vi "Motor Calibrator.vi"() -> ()   [LabVIEW 2013]
doc: "<B>Motor Control.vi</B> demonstrates simplistic control of a motor using PWM."
uses:
  <vilib>/Rock Robotics/SystemInterfaces/Typedef/FPGA_TypedefDigitalModule.ctl
  <vilib>/Rock Robotics/WPI/MotorControl/WPI_MotorControlOpen Victor.vi
  <vilib>/Rock Robotics/WPI/MotorControl/WPI_MotorControlOpen Jaguar.vi
  <vilib>/Rock Robotics/WPI/MotorControl/WPI_MotorControlOpen Talon.vi
panel:
  in  "Next":bool
  out "Current Motor":string="None"
  out "Motor Output":dbl(slide) scale=-1.0..1.0
  in  "Motor Controllers":cluster{"Type":u16, "PWM":string}[](array[cluster])=[{"Type"=0, "PWM"="PWM 1"}, {"Type"=0, "PWM"="PWM 2"}, {"Type"=0, "PWM"="PWM 3"}, {"Type"=0, "PWM"="PWM 4"}, {"Type"=0, "PWM"="PWM 5"}, {"Type"=0, "PWM"="PWM 6"}, {"Type"=0, "PWM"="PWM 7"}, {"Type"=0, "PWM"="PWM 8"}, {"Type"=0, "PWM"="PWM 9"}, {"Type"=0, "PWM"="PWM 10"}] {"Type" items=["Disabled", "Victor", "Jaguar", "Talon"]}
  in  "DIO Module":T1
  # "Calibration Instructions"
  # "Victor 888\n\n1. Power ON the speed controller.\n2. Press and hold the Cal button. After a moment, the LED indicator on the Victor will begin alternating between \n    RED and GREEN to indicate a cal mode.\n3. While continuing to hold the Cal button, move the joystick to the maximum and minimum positions. \n    This can be done in any order and as many times as desired.\n4. While continuing to hold the Cal button, return the joystick to center (neutral position).\n5. Release the Cal button.\n6. A flashing GREEN indicator confirms a successful calibration.\n7. A flashing RED indicator denotes an unsuccessful calibration.\n    An unsuccessful calibration occurs when either:\n    a) Insufficient joystick travel was detected in forward and/or reverse.\n    b) The trim tab is too far from center.\n    c) The Joystick is too far from center when Cal is released."
  # "Jaguar\n\n1. Hold down the USER switch with a straightened paper clip for 5 seconds.\n2. The LED flashes Red and Green to indicate Calibration mode.\n3. Instruct the controller to send a full-forward signal for one or more seconds.\n4. Instruct the controller to send a full-reverse signal for one or more seconds.\n5. The LED flashes Green and Yellow quickly to indicate a successful calibration."
  # "Talon\n\n1. Press and hold the button labeled “CAL” with a paper clip. The LED should begin to blink red/green. \n2. Continue to keep the button pressed while moving the joystick full forward and full reverse. \n    You may do this as many times as you like. \n3. Center the joystick and then release the CAL button. \n4. If calibration was successful, the LED will blink green several times. If the LED blinks red several times,\n    the calibration was not valid. If this happens, the Talon will use the last valid calibration values."
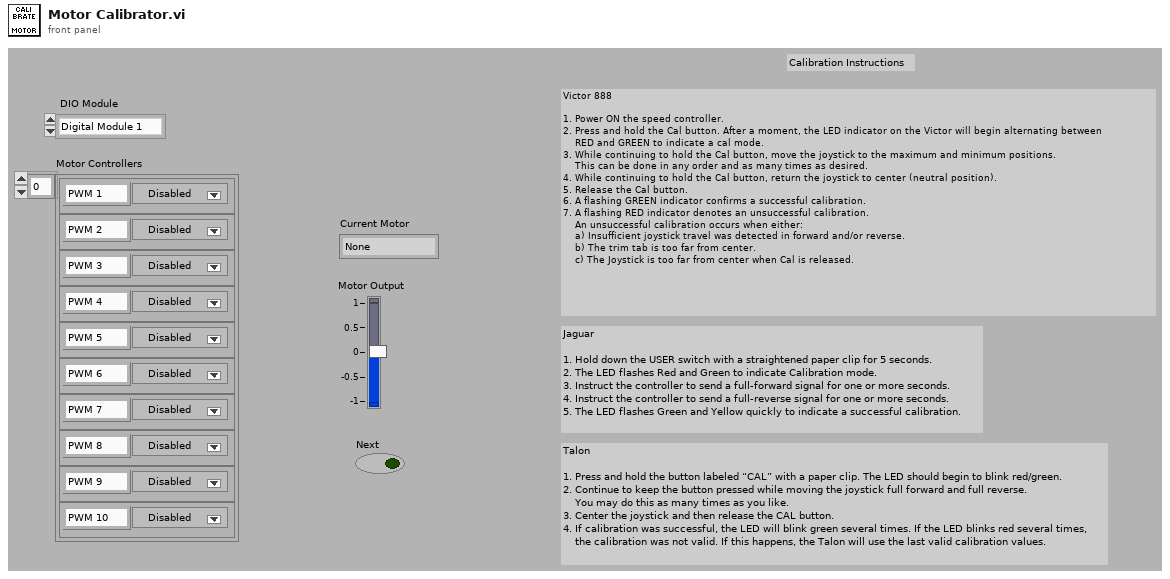
[diagram p1: front panel]
types:
  T1 = typedef "FPGA_TypedefDigitalModule.ctl" = enum16{"Digital Module 1", "Digital Module 2"}
  T2 = typedef "WPI_MotorControlDeviceRef.ctl" = cluster{"DeviceStatus":errorcluster, "Type":enum16{"PWM", "CAN"}, "PWM":cluster{"Digital Module":T1, "PWM Channel":T3, "DeadBand":T4}, "CAN":cluster{"Device Number":u8, "Control Mode":T5, "Semaphore":T6, "Max Vout":dbl}, "Invert":bool, "TransformRef":T7, "InvTransformRef":T7}
  T3 = typedef "FPGA_DIOPWMChannel.ctl" = enum8{"PWM 1", "PWM 2", "PWM 3", "PWM 4", "PWM 5", "PWM 6", "PWM 7", "PWM 8", "PWM 9", "PWM 10", "Invalid"}
  T4 = typedef "WPI_PWMDeadband.ctl" = cluster{"Name":string, "maxPositivePwm":i32, "minPositivePwm":i32, "centerPwm":i32, "maxNegativePwm":i32, "minNegativePwm":i32, "angularRange":u16}
  T5 = typedef "WPI_CANJaguar_ControlMode.ctl" = enum8{"Percent VBus", "Current", "Speed", "Position", "Voltage"}
  T6 = typedef "Semaphore RefNum" = refnum<k1>
  T7 = typedef "WPI_PWMTransform_ConPane.ctl" = refnum<vi>
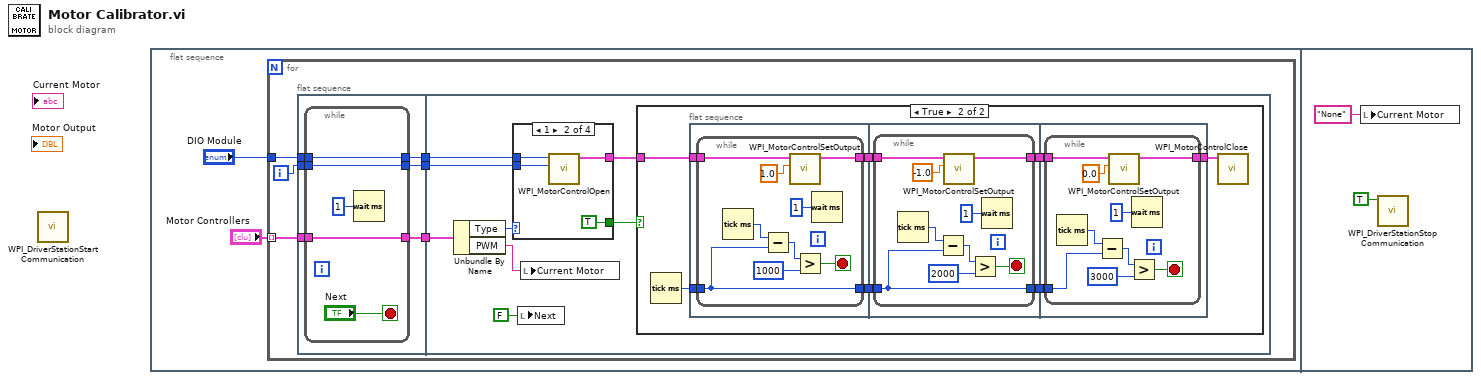
[diagram p0: block diagram]
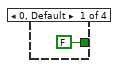
[diagram p3: hidden frame]
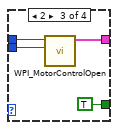
[diagram p4: hidden frame]
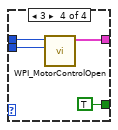
[diagram p5: hidden frame]
diagram:
  n1 = call <vilib>:"WPI_DriverStationStart Communication.vi"() -> ()  [unwired: 1 in, 11 out]
  n2 = flat-sequence {
    frame #0 {
      n3 = for {
        tunnel: "DIO Module" -> [w8]
        tunnel: "Motor Controllers" -> [w6] mode=indexing
        i -> [w7]
        n4 = flat-sequence {
          tunnel: w6 -> [w9]
          tunnel: w7 -> [w11]
          tunnel: w8 -> [w13]
          tunnel: [w14] -> w5
          tunnel: [w12] -> w4
          tunnel: [w10] -> w3
          tunnel: w5 -> [w26]
          tunnel: w4 -> [w25]
          tunnel: w3 -> [w24]
          frame #0 {
            n5 = while {
              tunnel: [w17] -> w14
              tunnel: w13 -> [w17]
              tunnel: [w16] -> w12
              tunnel: w11 -> [w16]
              tunnel: [w15] -> w10
              tunnel: w9 -> [w15]
              stop <- "Next" stop-if-true
              n6 = Wait (ms)(milliseconds to wait=u32 1) -> ()  [unwired: 1 out]
            }
          }
          frame #1 {
            n7 = Unbundle By Name(w24) -> ("Type"=w27:u16, "PWM"=w21:string)
            n8 = case shown="1" w27 {
              tunnel: w26 -> [_ w77 w81 w85]
              tunnel: w25 -> [_ w76 w80 w84]
              tunnel: [FALSE TRUE TRUE TRUE] -> w23
              tunnel: [_ w74 w78 w82] -> w22
              frame 0, Default {
              }
              frame 1 {
                n9 = call-poly <vilib>:"WPI_MotorControlOpen.vi"("PWM Channel"=w76, "Digital Module (Module 1)"=w77) -> ("MotorControlDeviceRef"=w74:T2)  [unwired: 5 in, 4 out]
              }
              frame 2 {
                n10 = call-poly <vilib>:"WPI_MotorControlOpen.vi"("PWM Channel"=w80, "Digital Module (Module 1)"=w81) -> ("MotorControlDeviceRef"=w78:T2)  [unwired: 5 in, 4 out]
              }
              frame 3 {
                n11 = call-poly <vilib>:"WPI_MotorControlOpen.vi"("PWM Channel"=w84, "Digital Module (Module 1)"=w85) -> ("MotorControlDeviceRef"=w82:T2)  [unwired: 5 in, 4 out]
              }
            }
            n12 = local write "Next"(FALSE ("Next")) -> ()
            n13 = local write "Current Motor"(w21) -> ()
            n14 = case shown="True" w23 {
              tunnel: w22 -> [_ w34]
              frame False {
              }
              frame True {
                n15 = Tick Count (ms)() -> (millisecond timer value=w30:u32)
                n16 = flat-sequence {
                  tunnel: [w38] -> w33
                  tunnel: w34 -> [w37]
                  tunnel: w30 -> [w36]
                  tunnel: [w35] -> w29
                  tunnel: [w51] -> w32
                  tunnel: w33 -> [w50]
                  tunnel: w29 -> [w49]
                  tunnel: [w48] -> w28
                  tunnel: [w63] -> w31
                  tunnel: w32 -> [w62]
                  tunnel: w28 -> [w61]
                  frame #0 {
                    n17 = while {
                      tunnel: [w47] -> w38
                      tunnel: w37 -> [w46]
                      tunnel: w36 -> [w40]
                      tunnel: [w40] -> w35
                      stop <- w44 stop-if-true
                      n18 = Tick Count (ms)() -> (millisecond timer value=w43:u32)
                      n19 = Subtract(x=w43, y=w40) -> (x-y=w42:u32)
                      n20 = call <vilib>:"WPI_MotorControlSetOutput.vi"("Output"=1.0, "MotorControlDevRef"=w46) -> ("MotorControlDevRef"=w47:T2)  [unwired: 3 in, 6 out]
                      n21 = Greater?(x=w42, y=u32 1000) -> (0:w44:bool)
                      n22 = Wait (ms)(milliseconds to wait=u32 1) -> ()  [unwired: 1 out]
                    }
                  }
                  frame #1 {
                    n23 = while {
                      tunnel: [w60] -> w51
                      tunnel: w50 -> [w59]
                      tunnel: w49 -> [w53]
                      tunnel: [w53] -> w48
                      stop <- w54 stop-if-true
                      n24 = Tick Count (ms)() -> (millisecond timer value=w57:u32)
                      n25 = Subtract(x=w57, y=w53) -> (x-y=w56:u32)
                      n26 = call <vilib>:"WPI_MotorControlSetOutput.vi"("Output"=-1.0, "MotorControlDevRef"=w59) -> ("MotorControlDevRef"=w60:T2)  [unwired: 3 in, 6 out]
                      n27 = Greater?(x=w56, y=u32 2000) -> (0:w54:bool)
                      n28 = Wait (ms)(milliseconds to wait=u32 1) -> ()  [unwired: 1 out]
                    }
                  }
                  frame #2 {
                    n29 = while {
                      tunnel: [w72] -> w63
                      tunnel: w62 -> [w71]
                      tunnel: w61 -> [w67]
                      stop <- w66 stop-if-true
                      n30 = Tick Count (ms)() -> (millisecond timer value=w70:u32)
                      n31 = Subtract(x=w70, y=w67) -> (x-y=w69:u32)
                      n32 = call <vilib>:"WPI_MotorControlSetOutput.vi"("Output"=0.0, "MotorControlDevRef"=w71) -> ("MotorControlDevRef"=w72:T2)  [unwired: 3 in, 6 out]
                      n33 = Greater?(x=w69, y=u32 3000) -> (0:w66:bool)
                      n34 = Wait (ms)(milliseconds to wait=u32 1) -> ()  [unwired: 1 out]
                    }
                  }
                }
                n35 = call <vilib>:"WPI_MotorControlClose.vi"("MotorControlDevRef"=w31) -> ()  [unwired: 1 in, 10 out]
              }
            }
          }
        }
      }
    }
    frame #1 {
      n36 = local write "Current Motor"("None" ("Current Motor")) -> ()
      n37 = call <vilib>:"WPI_DriverStationStop Communication.vi"("StopCommunication"=TRUE) -> ()  [unwired: 1 in, 10 out]
    }
  }
